vi "start-measurement-eventSD.vi"(1 "# current":refnum<vi>, 2 "NewVal":bool, 3 "cluster in":T1={"Kinetics"=[], "Spectrum"=[], "Experiments groups"=[], "GRAPH EXPERIMENTAL DATA"=[], "error out"={"status"=FALSE, "code"=0, "source"=""}, "group"=0, "exp selected"=0, "# exp"=0, "kinetics plot names"=[], "spectra plot names"=[], "FromToWave"={"FromWave"=0.0, "ToWave"=0.0}, "Laser shutter task"="", "Accelerator task"="", "Motor task"="", "GRAPH EXPERIMENTAL DATA ref"=refnum, "timedelays"=[0.0, 0.0, 0.0, 0.0, 0.0, 0.0, 0.0, 0.06019061100911815, 0.0521779104562645, 0.045231877429679615, 0.03921051490799832, 0.033990728811568754, 0.029465811603150715, 0.025543260876973825, 0.02214288834180205, 0.01919518054014414, 0.016639877791965713, 0.014424742312398925, 0.012504490320209958, 0.010839866306230088, 0.009396840537117498, 0.008145913389103785, 0.00706151229029317, 0.006121468943269439, 0.005306566140927374, 0.004600144911132549, 0.003987763959109073, 0.0034569044455719407, 0.00299671406541447, 0.0025977851951783253, 0.0022519625739982996, 0.00195217658646366, 0.0016922987392150965, 0.0014670163768006634, 0.0012717240756200802, 0.0011024294957352762, 0.0009556717658856477, 0.0008284507332614981, 0.0007181656316962257, 0.0006225619144775864, 0.0005396851648867825, 0.00046784114226338394, 0.0004055611468220084, 0.0003515719951773376, 0.00030476999279031153, 0.00026419837125694315, 0.00022902772919263772, 0.0001985390768670671, 0.0001721091379728629, 0.00014919760805372974, 0.00012933610911736794], "wavelengths"=[0.0, 0.0, 0.0, 0.0, 0.0, 0.0, 0.0, 0.06019061100911815, 0.0521779104562645, 0.045231877429679615, 0.03921051490799832, 0.033990728811568754, 0.029465811603150715, 0.025543260876973825, 0.02214288834180205, 0.01919518054014414, 0.016639877791965713, 0.014424742312398925, 0.012504490320209958, 0.010839866306230088, 0.009396840537117498, 0.008145913389103785, 0.00706151229029317, 0.006121468943269439, 0.005306566140927374, 0.004600144911132549, 0.003987763959109073, 0.0034569044455719407, 0.00299671406541447, 0.0025977851951783253, 0.0022519625739982996, 0.00195217658646366, 0.0016922987392150965, 0.0014670163768006634, 0.0012717240756200802, 0.0011024294957352762, 0.0009556717658856477, 0.0008284507332614981, 0.0007181656316962257, 0.0006225619144775864, 0.0005396851648867825, 0.00046784114226338394, 0.0004055611468220084, 0.0003515719951773376, 0.00030476999279031153, 0.00026419837125694315, 0.00022902772919263772, 0.0001985390768670671, 0.0001721091379728629, 0.00014919760805372974, 0.00012933610911736794], "Experiment"=refnum, "Commentaires exp"=refnum, "FromToDelay"={"FromDelay"=0.0, "ToDelay"=0.0}}, 4 "Measure event":refnum<user-event>, 5 "notifier mesure in":refnum<notifier>) -> (0 "cluster out":T1={"Kinetics"=[], "Spectrum"=[], "Experiments groups"=[], "GRAPH EXPERIMENTAL DATA"=[], "error out"={"status"=FALSE, "code"=0, "source"=""}, "group"=0, "exp selected"=0, "# exp"=0, "kinetics plot names"=[], "spectra plot names"=[], "FromToWave"={"FromWave"=0.0, "ToWave"=0.0}, "Laser shutter task"="", "Accelerator task"="", "Motor task"="", "GRAPH EXPERIMENTAL DATA ref"=refnum, "timedelays"=[0.0, 0.0, 0.0, 0.0, 0.0, 0.0, 0.0, 0.06019061100911815, 0.0521779104562645, 0.045231877429679615, 0.03921051490799832, 0.033990728811568754, 0.029465811603150715, 0.025543260876973825, 0.02214288834180205, 0.01919518054014414, 0.016639877791965713, 0.014424742312398925, 0.012504490320209958, 0.010839866306230088, 0.009396840537117498, 0.008145913389103785, 0.00706151229029317, 0.006121468943269439, 0.005306566140927374, 0.004600144911132549, 0.003987763959109073, 0.0034569044455719407, 0.00299671406541447, 0.0025977851951783253, 0.0022519625739982996, 0.00195217658646366, 0.0016922987392150965, 0.0014670163768006634, 0.0012717240756200802, 0.0011024294957352762, 0.0009556717658856477, 0.0008284507332614981, 0.0007181656316962257, 0.0006225619144775864, 0.0005396851648867825, 0.00046784114226338394, 0.0004055611468220084, 0.0003515719951773376, 0.00030476999279031153, 0.00026419837125694315, 0.00022902772919263772, 0.0001985390768670671, 0.0001721091379728629, 0.00014919760805372974, 0.00012933610911736794], "wavelengths"=[0.0, 0.0, 0.0, 0.0, 0.0, 0.0, 0.0, 0.06019061100911815, 0.0521779104562645, 0.045231877429679615, 0.03921051490799832, 0.033990728811568754, 0.029465811603150715, 0.025543260876973825, 0.02214288834180205, 0.01919518054014414, 0.016639877791965713, 0.014424742312398925, 0.012504490320209958, 0.010839866306230088, 0.009396840537117498, 0.008145913389103785, 0.00706151229029317, 0.006121468943269439, 0.005306566140927374, 0.004600144911132549, 0.003987763959109073, 0.0034569044455719407, 0.00299671406541447, 0.0025977851951783253, 0.0022519625739982996, 0.00195217658646366, 0.0016922987392150965, 0.0014670163768006634, 0.0012717240756200802, 0.0011024294957352762, 0.0009556717658856477, 0.0008284507332614981, 0.0007181656316962257, 0.0006225619144775864, 0.0005396851648867825, 0.00046784114226338394, 0.0004055611468220084, 0.0003515719951773376, 0.00030476999279031153, 0.00026419837125694315, 0.00022902772919263772, 0.0001985390768670671, 0.0001721091379728629, 0.00014919760805372974, 0.00012933610911736794], "Experiment"=refnum, "Commentaires exp"=refnum, "FromToDelay"={"FromDelay"=0.0, "ToDelay"=0.0}})   [LabVIEW 2015]
uses:
  controls/control-cluster.ctl
  Classes/Experiments_group.lvclass
  Classes/Experiment.lvclass
  globalVarSD.vi
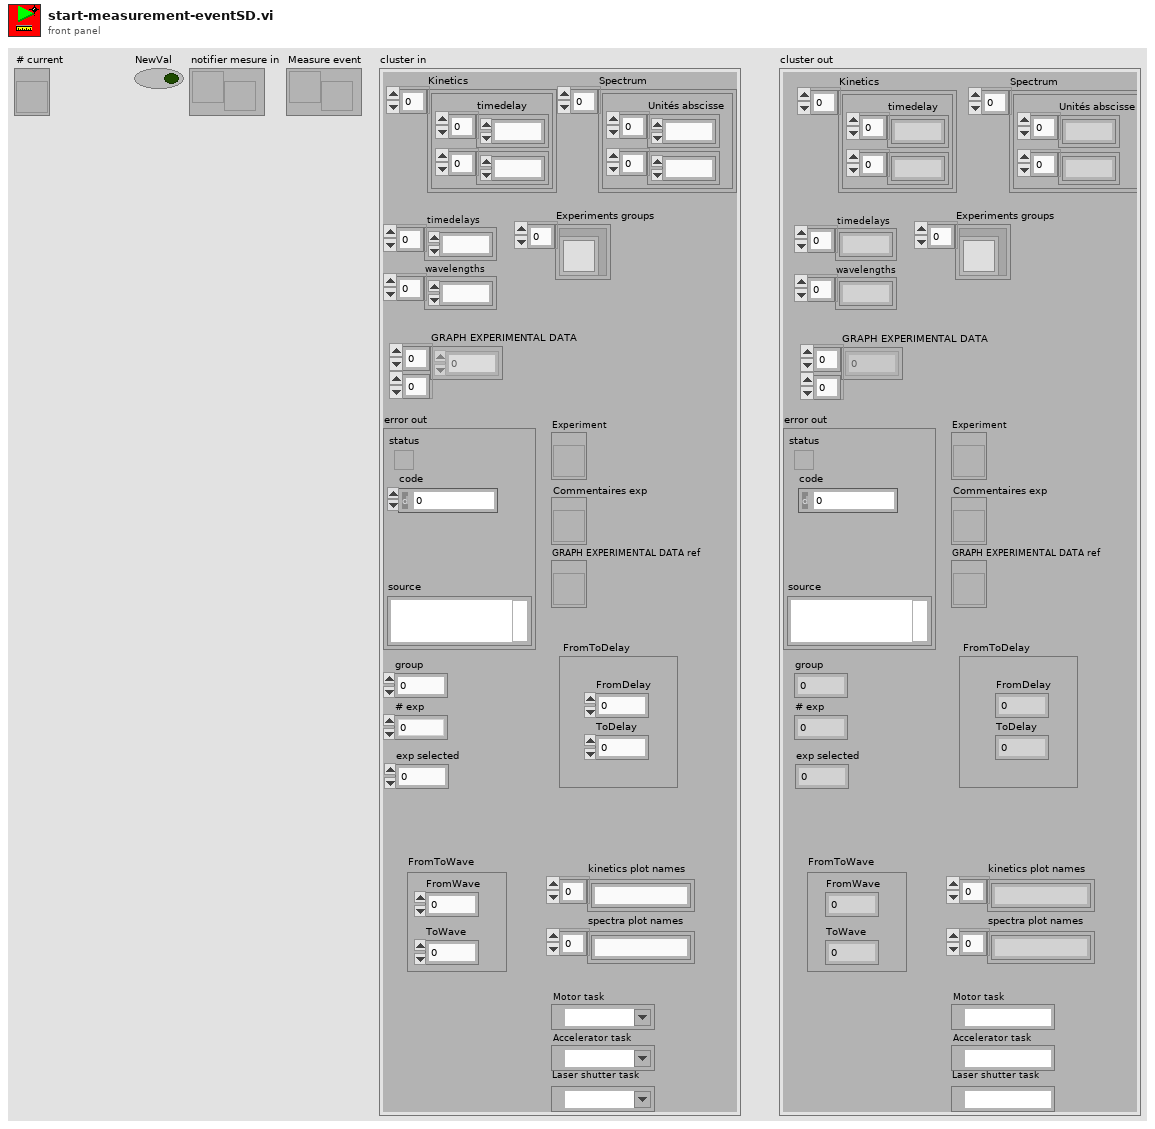
[diagram p1: front panel]
types:
  T1 = typedef "control-cluster.ctl" = cluster{"Kinetics":cluster{"timedelay":dbl[], dbl[]}[], "Spectrum":cluster{"Unités abscisse":dbl[], dbl[]}[], "Experiments groups":refnum<class "Experiments_group.lvclass">[], "GRAPH EXPERIMENTAL DATA":dbl[][], "error out":errorcluster, "group":i32, "exp selected":i32, "# exp":i32, "kinetics plot names":string[], "spectra plot names":string[], "FromToWave":cluster{"FromWave":dbl, "ToWave":dbl}, "Laser shutter task":refnum<k21>, "Accelerator task":refnum<k21>, "Motor task":refnum<k21>, "GRAPH EXPERIMENTAL DATA ref":refnum<vi>, "timedelays":dbl[], "wavelengths":dbl[], "Experiment":refnum<vi>, "Commentaires exp":refnum<vi>, "FromToDelay":cluster{"FromDelay":dbl, "ToDelay":dbl}}
  T2 = enum8{"Enabled", "Disabled", "Disabled and Grayed Out"}
  T3 = cluster{bool, "Experiment.lvclass out":refnum<class "Experiment.lvclass">, path}
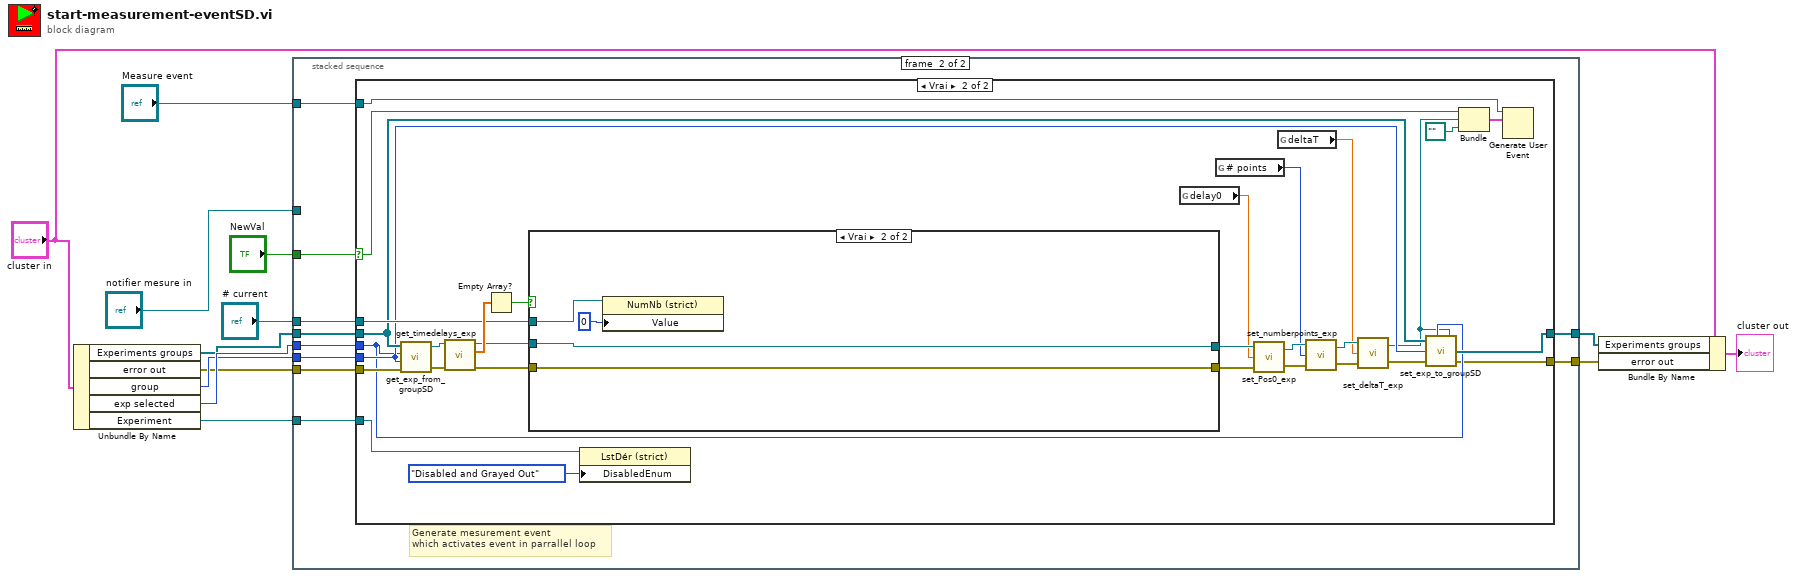
[diagram p0: block diagram]
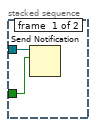
[diagram p2: hidden frame]
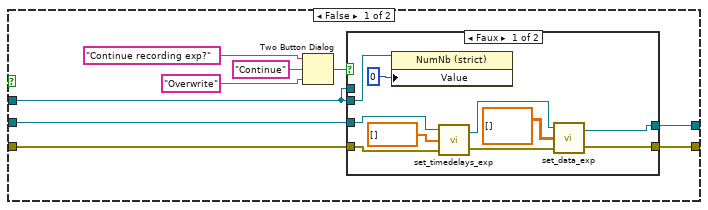
[diagram p4: hidden frame]
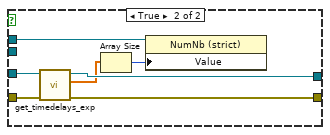
[diagram p5: hidden frame]
diagram:
  n1 = Unbundle By Name("cluster in") -> ("Experiments groups"=w9:refnum<class "Experiments_group.lvclass">[], "error out"=w10:errorcluster, "group"=w12:i32, "exp selected"=w13:i32, "Experiment"=w1:refnum<vi>)
  n2 = stacked-sequence {
    tunnel: "notifier mesure in" -> [w15 _]
    tunnel: "Measure event" -> [_ w25]
    tunnel: "NewVal" -> [w14 w24]
    tunnel: [_ w23] -> w11
    tunnel: w9 -> [_ w22]
    tunnel: w10 -> [_ w21]
    tunnel: w12 -> [_ w20]
    tunnel: w13 -> [_ w19]
    tunnel: w1 -> [_ w18]
    tunnel: "# current" -> [_ w17]
    tunnel: [_ w16] -> w2
    frame #0 {
      n3 = Send Notification(notification=w14, notifier=w15) -> ()  [unwired: 1 in, 2 out]
    }
    frame #1 {
      # "Generate mesurement event\nwhich activates event in parrallel loop"
      n4 = case shown="Vrai" w24 {
        selector: w24 -> [_ w31]
        tunnel: w25 -> [_ w57]
        tunnel: [w27 w32] -> w23
        tunnel: w22 -> [w26 w38]
        tunnel: w21 -> [w27 w48]
        tunnel: w20 -> [_ w36]
        tunnel: w19 -> [_ w35]
        tunnel: w18 -> [_ w47]
        tunnel: w17 -> [_ w46]
        tunnel: [w26 w37] -> w16
        frame False {
        }
        frame True {
          n5 = call "get_exp_from_groupSD.vi"("error in (no error)"=w48, "group"=w36, "exp selected"=w35, "Experiments groups"=w38) -> ("error out"=w49:errorcluster, "Experiment out"=w50:refnum<class "Experiment.lvclass">)  [unwired: 1 out]
          n6 = call-dynamic "get_timedelays_exp.vi"("error in (no error)"=w49, "Experiment.lvclass in"=w50) -> ("error out"=w51:errorcluster, "timedelays"=w54:dbl[], "Experiment.lvclass out"=w52:refnum<class "Experiment.lvclass">)  [unwired: 7 in]
          n7 = Empty Array?(array=w54) -> (empty?=w53:bool)
          n8 = case shown="Vrai" w53 {
            tunnel: [w61 w87] -> w42
            tunnel: w52 -> [w62 w87]
            tunnel: w51 -> [w60 w86]
            tunnel: [w59 w86] -> w41
            tunnel: w46 -> [w58 w85]
            frame False {
              n9 = Two Button Dialog(message="Continue recording exp?", 1:"Overwrite" ("F button name (\"Cancel\")"), 2:"Continue" ("T button name (\"OK\")")) -> (T button?=w63:bool)
              n10 = case shown="Faux" w63 {
                tunnel: w62 -> [w73 w83]
                tunnel: [w71 w82] -> w61
                tunnel: w60 -> [w74 w80]
                tunnel: [w69 w79] -> w59
                tunnel: w58 -> [w67 _]
                tunnel: w58 -> [_ w77]
                frame False {
                  n11 = property class="NumNb (strict)"(reference=w67, "Value"=0 ("#")) -> ()  [unwired: 1 in, 2 out]
                  n12 = call-dynamic "set_timedelays_exp.vi"("error in (no error)"=w74, "timedelays"=dbl[] [], "Experiment.lvclass in"=w73) -> ("error out"=w70:errorcluster, "Experiment.lvclass out"=w72:refnum<class "Experiment.lvclass">)
                  n13 = call-dynamic "set_data_exp.vi"("error in (no error)"=w70, "Data"=dbl[][] [], "Experiment.lvclass in"=w72) -> ("error out"=w69:errorcluster, "Experiment.lvclass out"=w71:refnum<class "Experiment.lvclass">)
                }
                frame True {
                  n14 = call-dynamic "get_timedelays_exp.vi"("error in (no error)"=w80, "Experiment.lvclass in"=w83) -> ("error out"=w79:errorcluster, "timedelays"=w78:dbl[], "Experiment.lvclass out"=w82:refnum<class "Experiment.lvclass">)  [unwired: 7 in]
                  n15 = Array Size(array=w78) -> (size(s)=w81:i32)
                  n16 = property class="NumNb (strict)"(reference=w77, "Value"=w81) -> ()  [unwired: 1 in, 2 out]
                }
              }
            }
            frame True {
              n17 = property class="NumNb (strict)"(reference=w85, "Value"=0) -> ()  [unwired: 1 in, 2 out]
            }
          }
          n18 = property on="Property Node" class="LstDér (strict)"(reference=w47, "DisabledEnum"=T2."Disabled and Grayed Out" ("Disabled")) -> ()  [unwired: 1 in, 2 out]
          n19 = global read "globalVarSD.vi" "delay0"() -> (w28:dbl)
          n20 = global read "globalVarSD.vi" "# points"() -> (w29:i32)
          n21 = call-dynamic "set_Pos0_exp.vi"("error in (no error)"=w41, "Pos0,ps"=w28, "Experiment.lvclass in"=w42) -> ("error out"=w40:errorcluster, "Experiment.lvclass out"=w43:refnum<class "Experiment.lvclass">)
          n22 = global read "globalVarSD.vi" "deltaT"() -> (w30:dbl)
          n23 = call-dynamic "set_numberpoints_exp.vi"("error in (no error)"=w40, "numberpoints"=w29, "Experiment.lvclass in"=w43) -> ("error out"=w39:errorcluster, "Experiment.lvclass out"=w44:refnum<class "Experiment.lvclass">)
          n24 = call-dynamic "set_deltaT_exp.vi"("error in (no error)"=w39, "deltaTlast"=w30, "Experiment.lvclass in"=w44) -> ("error out"=w33:errorcluster, "Experiment.lvclass out"=w34:refnum<class "Experiment.lvclass">)
          n25 = call "set_exp_to_groupSD.vi"("Experiments groups"=w38, "exp selected"=w35, "group"=w36, "error in (no error)"=w33, "Experiment in"=w34) -> ("Experiments groups out"=w37:refnum<class "Experiments_group.lvclass">[], "error out"=w32:errorcluster)  [unwired: 1 in]
          n26 = Bundle(w31, "Experiment.lvclass out"=w34, path "") -> (w56:T3)  [unwired: 1 in]
          n27 = Generate User Event(user event=w57, event data cluster=w56) -> ()  [unwired: 2 in, 2 out]
        }
      }
    }
  }
  n28 = Bundle By Name(cluster="cluster in", "Experiments groups"=w2, "error out"=w11) -> (→"cluster out":T1)
